vi "GetTargetIPAddresses.vi"(8 "error in (no error)":errorcluster, 11 "absolute system definition file":path) -> (0 "error out":errorcluster, 3 "ip addresses":string[](array[string]))   [LabVIEW 2015, in "VeriStandTestCase.lvclass"]
uses:
  VeriStandTestCase.lvclass
  <vilib>/xml/Load XML File.vi
  <vilib>/xml/Close Reference(Node).vi
  <vilib>/xml/NI_XML.lvlib
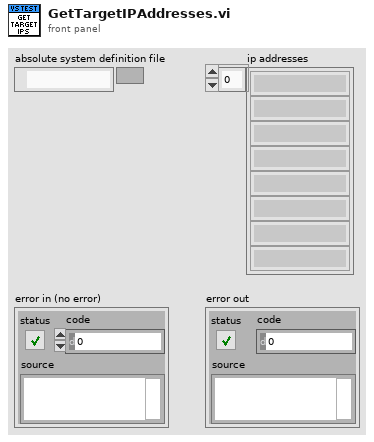
[diagram p1: front panel]
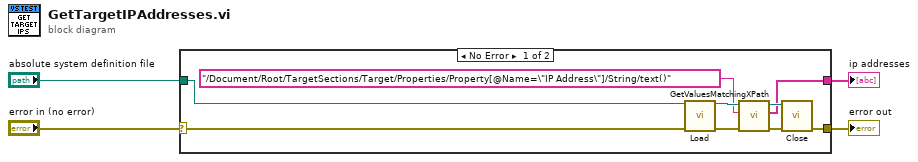
[diagram p0: block diagram]
diagram:
  n1 = case shown="No Error" "error in (no error)" {
    selector: "error in (no error)" -> [w13 w14]
    tunnel: [w12 w14] -> w3
    tunnel: "absolute system definition file" -> [w11 _]
    tunnel: [w6 _] -> w1
    frame No Error {
      n2 = call-poly <vilib>:"Load.vi"("path to XML document"=w11, "error in (no error)"=w13) -> ("DOM document out"=w7:refnum<k20>, "error out"=w8:errorcluster)  [unwired: 11 in, 1 out]
      n3 = call "GetValuesMatchingXPath.vi"("error in (no error)"=w8, "XPath"="/Document/Root/TargetSections/Target/Properties/Property[@Name=\"IP Address\"]/String/text()", "XML refnum in"=w7) -> ("error out"=w9:errorcluster, "Values"=w6:string[], "XML refnum out"=w10:refnum<k20>)  [unwired: 6 in]
      n4 = call-poly <vilib>:"Close.vi"("error in (no error)"=w9, "node"=w10) -> ("error out"=w12:errorcluster)  [unwired: 7 in]
    }
    frame Error {
    }
  }
  "error out" <- w3
  "ip addresses" <- w1
